vi "Assignment W1.vi"() -> ()   [LabVIEW 2017]
panel:
  in  "String":string
  out "Kilometer per hour":dbl
  in  "Mile per hour":dbl
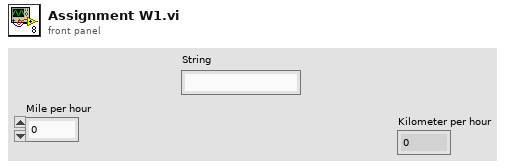
[diagram p1: front panel]
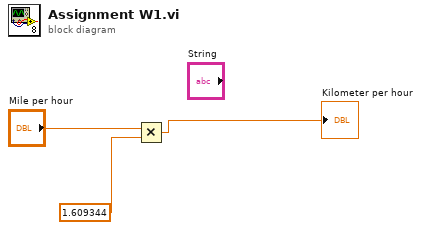
[diagram p0: block diagram]
diagram:
  n1 = Multiply(x="Mile per hour", y=1.609344) -> (x*y=→"Kilometer per hour":dbl)
